vi "Position From The Target.vi"(0 "Distance Left":dbl, 1 "alpha tag":dbl, 2 "Distance Right":dbl, 3 "X":dbl, 4 "beta tag":dbl) -> (5 "Delta X":dbl, 6 "Delta Y":dbl)   [LabVIEW 2016]
panel:
  out "Gama":dbl
  out "Theta":dbl
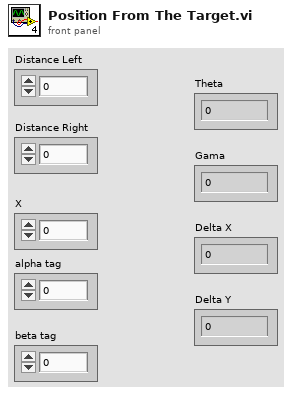
[diagram p1: front panel]
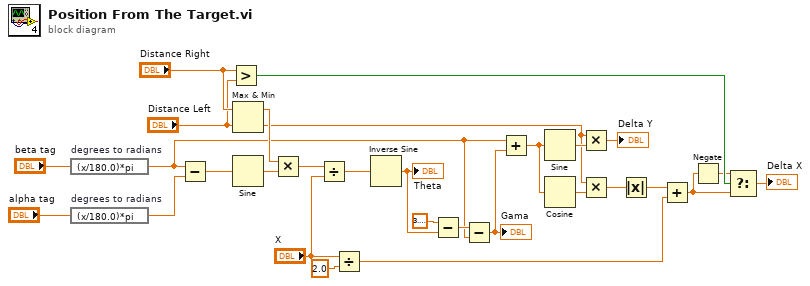
[diagram p0: block diagram]
diagram:
  n1 = expression code="(x/180.0)*pi" "degrees to radians"("beta tag") -> (w11:dbl)
  n2 = expression code="(x/180.0)*pi" "degrees to radians"("alpha tag") -> (w10:dbl)
  n3 = Subtract(x=w11, y=w10) -> (x-y=w29:dbl)
  n4 = Greater?(x="Distance Right", y="Distance Left") -> (0:w6:bool)
  n5 = Max & Min(x="Distance Right", y="Distance Left") -> (max(x,y)=w13:dbl, min(x,y)=w12:dbl)
  n6 = Sine(x=w29) -> (sin(x)=w28:dbl)
  n7 = Multiply(x=w13, y=w28) -> (x*y=w27:dbl)
  n8 = Divide(x=w27, y="X") -> (x/y=w26:dbl)
  n9 = Divide(x="X", y=2.0) -> (x/y=w21:dbl)
  n10 = Inverse Sine(1:w26) -> (0:w8:dbl)
  "Theta" <- w8
  n11 = Subtract(x=3.141592653589793, y=w8) -> (x-y=w25:dbl)
  n12 = Subtract(x=w25, y=w11) -> (x-y=w24:dbl)
  "Gama" <- w24
  n13 = Add(x=w11, y=w24) -> (x+y=w18:dbl)
  n14 = Sine(x=w18) -> (sin(x)=w17:dbl)
  n15 = Cosine(x=w18) -> (cos(x)=w20:dbl)
  n16 = Multiply(x=w12, y=w17) -> (x*y=→"Delta Y":dbl)
  n17 = Multiply(x=w12, y=w20) -> (x*y=w19:dbl)
  n18 = Absolute Value(x=w19) -> (abs(x)=w7:dbl)
  n19 = Add(x=w7, y=w21) -> (x+y=w1:dbl)
  n20 = Negate(x=w1) -> (-x=w2:dbl)
  n21 = Select(t=w2, s=w6, f=w1) -> (s? t:f=→"Delta X":dbl)
